vi "Config Part Type.vi"() -> ()   [LabVIEW 2018]
uses:
  05.UserVI's/type defs/EOL Part Setup.ctl
  02.Type Def's/All Communication Types.ctl
  05.UserVI's/type defs/Communication with Motors.ctl
  05.UserVI's/type defs/RAP Signal Control.ctl
  05.UserVI's/type defs/EOL Motor Type.ctl
panel:
  in  "Array":T1[](array[typedef])=[{"Communication Type"=enum."RS 232 LIN", "Send Messages to"=enum."Glass", "RAP Signal"=enum."High", "Motor Type"=enum."Smart Motor", "NVH Part Number"=0, "Turn Off Timer"=0, "Part Type"="C5"}, {"Communication Type"=enum."RS 232 LIN", "Send Messages to"=enum."Glass", "RAP Signal"=enum."High", "Motor Type"=enum."Smart Motor", "NVH Part Number"=0, "Turn Off Timer"=0, "Part Type"="C520"}]
  in  "Exit":bool
  in  "Save":bool
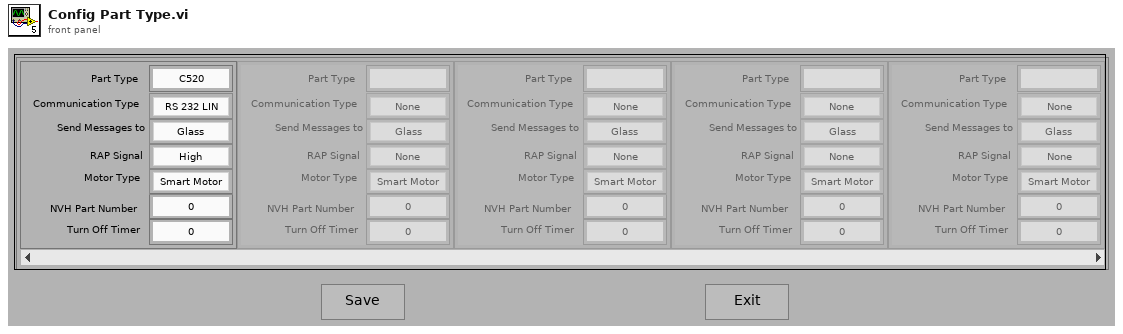
[diagram p1: front panel]
types:
  T1 = typedef "EOL Part Setup.ctl" = cluster{"Communication Type":T2, "Send Messages to":T3, "RAP Signal":T4, "Motor Type":T5, "NVH Part Number":u16, "Turn Off Timer":u16, "Part Type":string}
  T2 = typedef "All Communication Types.ctl" = enum16{"None", "CAN", "RS 232", "RS 232 LIN", "GM LIN", "SnT LIN", "K Line", "Robel CAN", "P42M-Continental", "Inalfa SCU LIN", "Spare 3"}
  T3 = typedef "Communication with Motors.ctl" = enum16{"Glass", "Rollo", "Both"}
  T4 = typedef "RAP Signal Control.ctl" = enum16{"High", "Low", "None"}
  T5 = typedef "EOL Motor Type.ctl" = enum16{"Smart Motor", "Sensor Motor"}
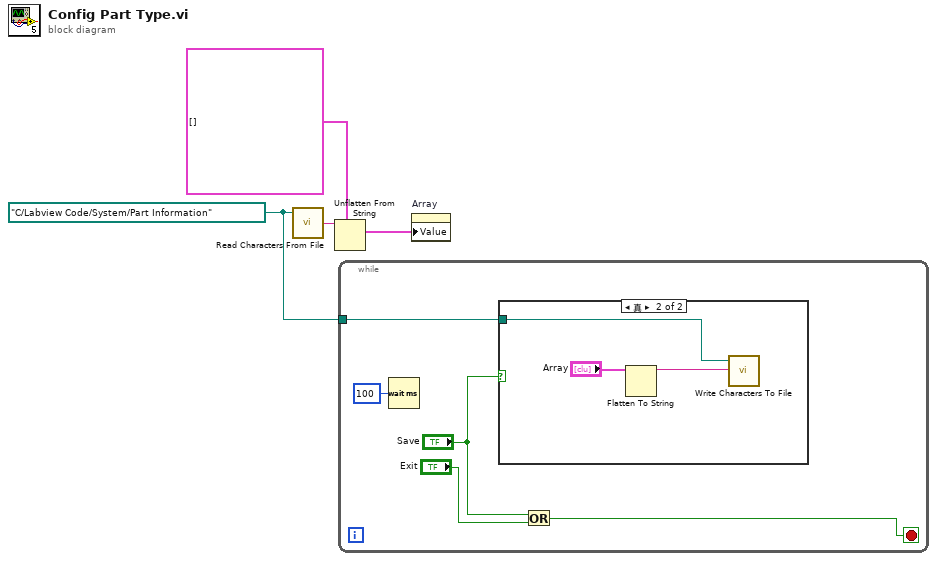
[diagram p0: block diagram]
diagram:
  w2 = path "C:/Labview Code/System/Part Information" ("file path (dialog if empty)")
  n1 = call <vilib>:"Read Characters From File.vi"("file path (dialog if empty)"=w2) -> ("character string"=w4:string)  [unwired: 5 in, 3 out]
  n2 = Unflatten From String(type=T1[] [] ("Array"), binary string=w4) -> (value=w1:T1[])  [unwired: 3 in, 2 out]
  n3 = while {
    tunnel: w2 -> [w6]
    stop <- w8 stop-if-true
    n4 = Wait (ms)(milliseconds to wait=u32 100) -> ()  [unwired: 1 out]
    n5 = case shown="真" "Save" {
      tunnel: w6 -> [_ w11]
      frame False {
      }
      frame True {
        n6 = Flatten To String(anything="Array") -> (data string=w12:string)  [unwired: 3 in, 2 out]
        n7 = call <vilib>:"Write Characters To File.vi"("character string"=w12, "file path (dialog if empty)"=w11) -> ()  [unwired: 3 in, 1 out]
      }
    }
    n8 = Or(x="Save", y="Exit") -> (x .or. y?=w8:bool)
  }
  n9 = property on="Array" class="Arr (严格)"("Value"=w1) -> ()  [unwired: 2 in, 2 out]
